vi "Autonics_Speed.vi"(5 "Multiplier":dbl=10.0, 7 "Speed (mm/s)":dbl=10.0, 8 "error in (no error)":errorcluster, 10 "Travel per  Pulse":dbl=0.002, 11 "VISA resource name":refnum<visa-resource-name>) -> (0 "error out":errorcluster, 3 "VISA resource name out":refnum<visa-resource-name>)   [LabVIEW 2018]
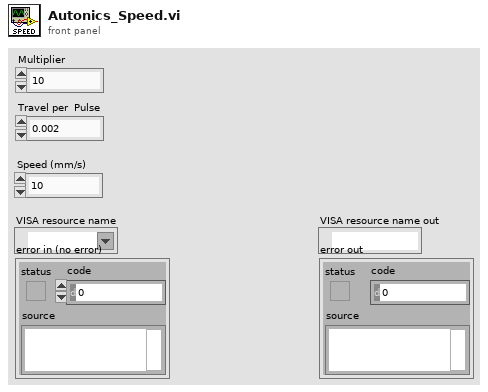
[diagram p1: front panel]
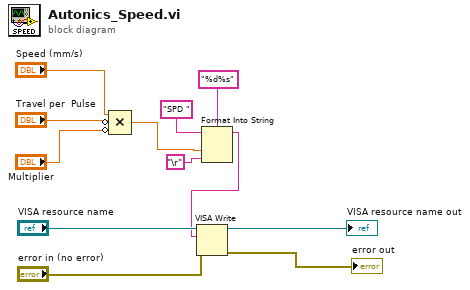
[diagram p0: block diagram]
diagram:
  n1 = Compound Arithmetic op=MULTIPLY("Speed (mm/s)", invert "Travel per  Pulse", invert "Multiplier") -> (w8:dbl)
  n2 = Format Into String(format string="%d%s", initial string="SPD " ("string"), w8, "\r") -> (resulting string=w1:string)  [unwired: 1 in, 1 out]
  n3 = VISA Write(VISA resource name="VISA resource name", write buffer=w1, error in (no error)="error in (no error)") -> (VISA resource name out=→"VISA resource name out":refnum<visa-resource-name>, error out=→"error out":errorcluster)  [unwired: 1 out]
